vi "LinearPlntInvFF_Reset_Zero.vi"(11 "Input Linear Plant Inv FF":T1) -> (3 "Output Linear Plant Inv FF":T1)   [LabVIEW 2019, in "Trajectory_Library.lvlib"]
doc: "Resets the feedforward with a zero initial state vector. \n\nInputs:\n - LinearPlntInversionFF -- system data cluster\n\nOutputs:\n - outLinearPlntInversionFF -- updated system data cluster"
uses:
  Trajectory_Library.lvlib
  TypeDef/LINEAR_PLANT_INV_FF.ctl
  <vilib>/Analysis/Matrix/Datatypes/RealMatrix.ctl
  <vilib>/Analysis/Matrix/NI_Matrix.lvlib
panel:
  # "<States,1>"
  # "<Inputs,1>"
  # "<States,Inputs>"
  # "<States,States>"
  # "<States,1>"
  # "<Inputs,1>"
  # "<States,Inputs>"
  # "<States,States>"
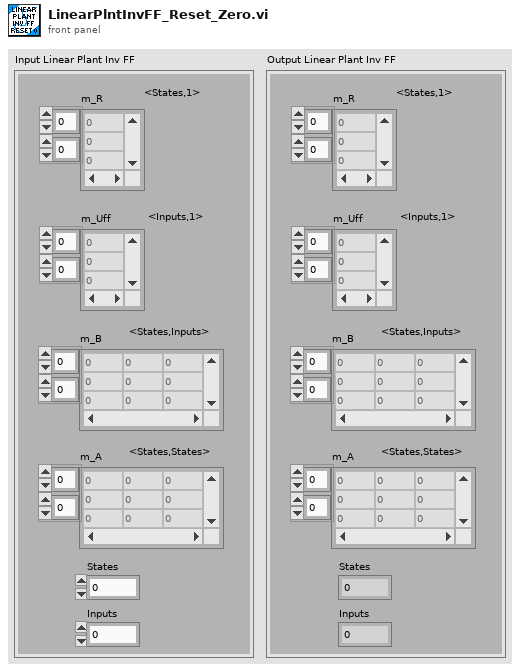
[diagram p1: front panel]
types:
  T1 = typedef "Trajectory_Library.lvlib/LINEAR_PLANT_INV_FF.ctl" = cluster{"m_R":T2, "m_Uff":T2, "m_B":T2, "m_A":T2, "States":i32, "Inputs":i32}
  T2 = typedef "NI_Matrix.lvlib/RealMatrix.ctl" = dbl[][]
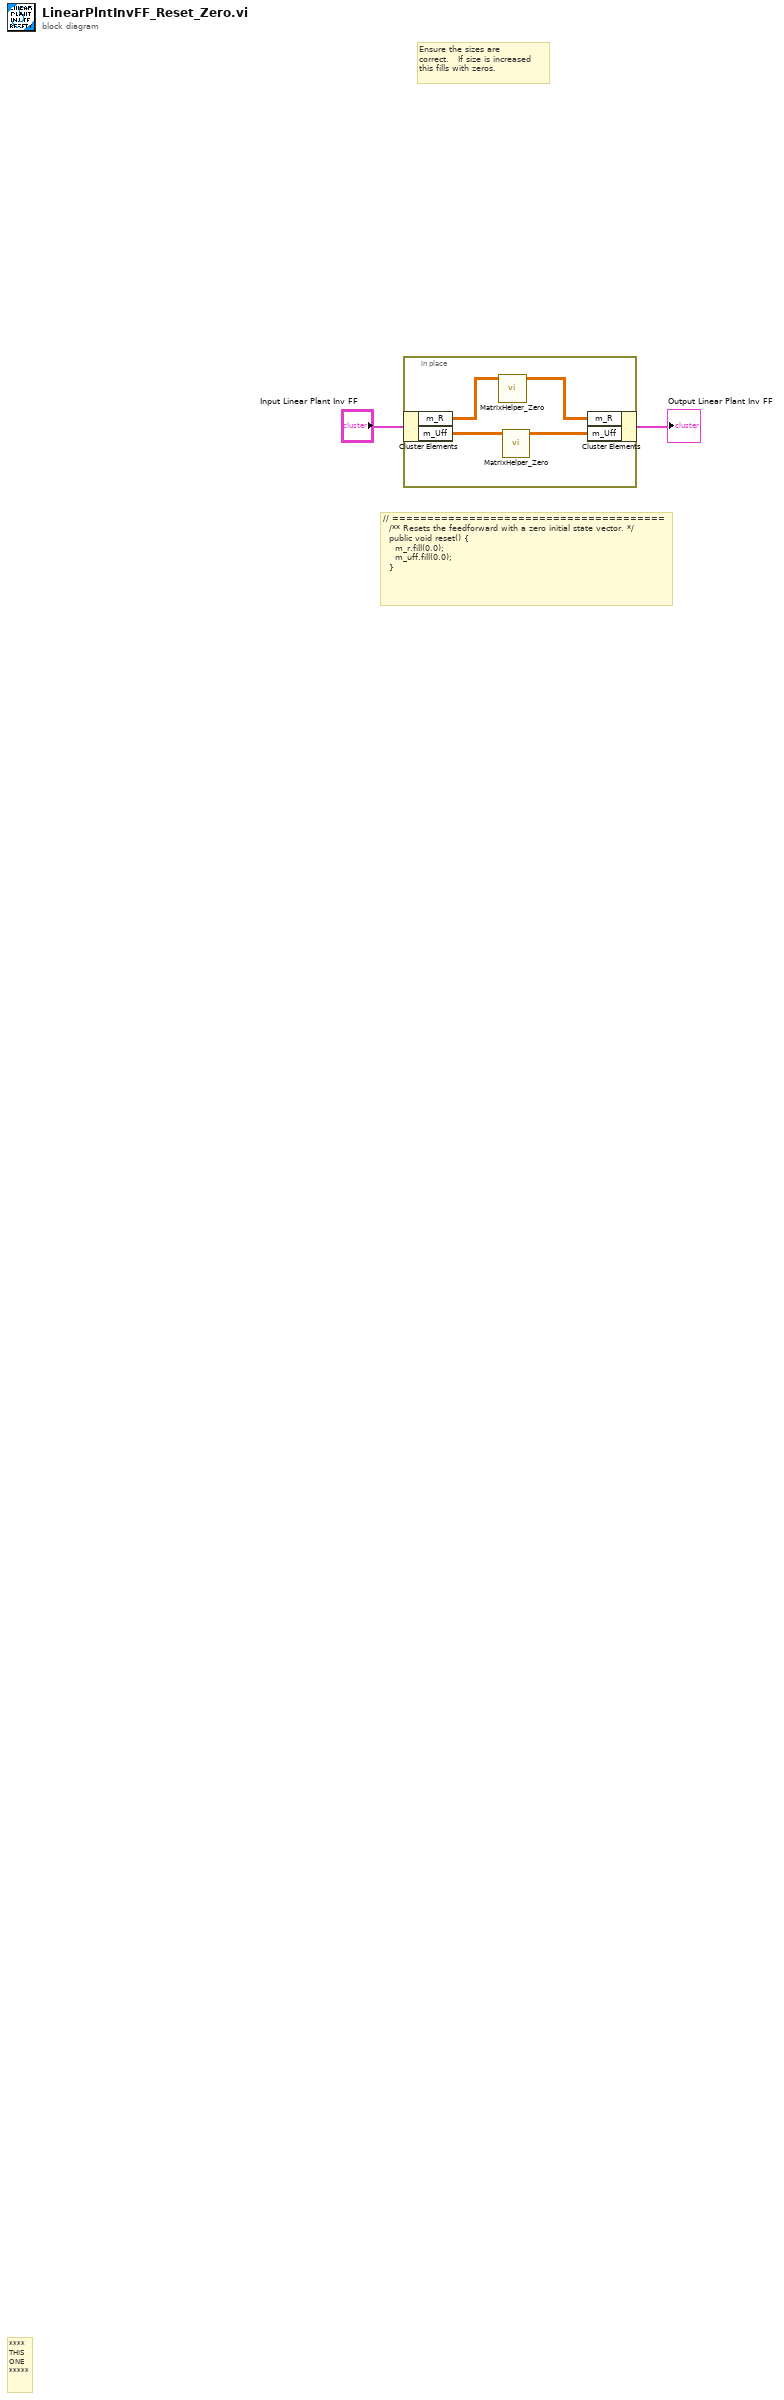
[diagram p0: block diagram]
diagram:
  # "// =======================================\n  /** Resets the feedforward with a zero initial state vector. */\n  public void reset() {\n    m_r.fill(0.0);\n    m_uff.fill(0.0);\n  }"
  # "Ensure the sizes are\ncorrect.   If size is increased \nthis fills with zeros."
  # "****\nTHIS\nONE\n*****"
  n1 = in-place {
    n2 = in-place-cluster #1("Input Linear Plant Inv FF") -> ("m_R"=w6:T2, "m_Uff"=w4:T2)
    n3 = call "MatrixHelper_Zero.vi"("input matrix"=w6) -> ("output matrix"=w5:T2)  [unwired: 10 in]
    n4 = call "MatrixHelper_Zero.vi"("input matrix"=w4) -> ("output matrix"=w3:T2)  [unwired: 10 in]
    n5 = in-place-cluster #1("m_R"=w5, "m_Uff"=w3) -> (→"Output Linear Plant Inv FF":T1)
  }
